vi "Read Boolean Variable.vi"(2 "error in (no error)":errorcluster, 3 "Name":string) -> (0 "error out":errorcluster, 1 "Value":bool)   [LabVIEW 2014]
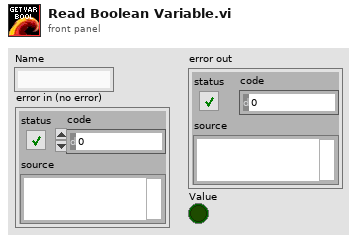
[diagram p1: front panel]
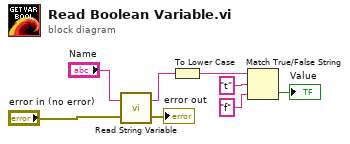
[diagram p0: block diagram]
diagram:
  n1 = call "Read String Variable.vi"("error in (no error)"="error in (no error)", "Name"="Name") -> ("error out"=→"error out":errorcluster, "Variable"=w3:string)
  n2 = To Lower Case(string=w3) -> (all lower case string=w2:string)
  n3 = Match True/False String(2:"f" ("false string"), 3:"t" ("true string"), 4:w2) -> (0:→"Value":bool)  [unwired: 1 out]
